vi "create GWS access config.vi"(4 "error in (no error)":errorcluster) -> (0 "error out":errorcluster)   [LabVIEW 2011]
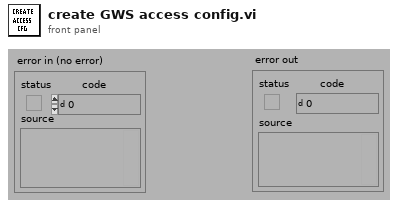
[diagram p1: front panel]
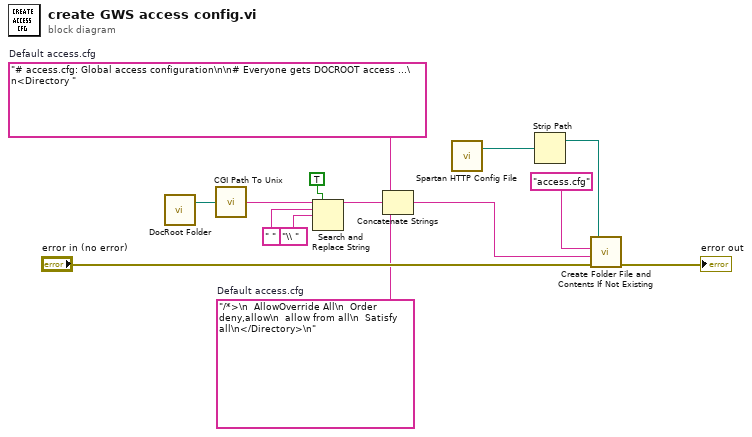
[diagram p0: block diagram]
diagram:
  w8 = "/*>\n  AllowOverride All\n  Order deny,allow\n  allow from all\n  Satisfy all\n</Directory>\n"  # Default access.cfg
  w9 = "# access.cfg: Global access configuration\n\n# Everyone gets DOCROOT access ...\n<Directory "  # Default access.cfg
  n1 = call "DocRoot Folder.vi"() -> ("DocumentRoot Folder"=w1:path)  [unwired: 3 in]
  n2 = call "CGI Path To Unix.vi"("platform path"=w1) -> ("unix path"=w3:string)  [unwired: 1 in]
  n3 = Search and Replace String(replace all?=TRUE ("replace all? (F)"), input string=w3, search string=" ", replace string="\\ " ("replace string (\"\")")) -> (result string=w2:string)  [unwired: 1 in, 6 out]
  n4 = Concatenate Strings(w9, w2, w8) -> (w7:string)
  n5 = call "Spartan HTTP Config File.vi"() -> ("HTTP Configuration File"=w11:path)  [unwired: 1 out]
  n6 = Strip Path(path=w11) -> (stripped path=w10:path)  [unwired: 1 out]
  n7 = call "Create Folder File and Contents If Not Existing.vi"("error in (no error)"="error in (no error)", "File contents to write (\"\")"=w7, "Filename (\"\")"="access.cfg", "File Folder (Empty)"=w10) -> ("error out"=→"error out":errorcluster)  [unwired: 3 out]
